vi "Counts Per Second to RPM.vi"(10 "Counts/Rev":dbl, 11 "Counts/Second":dbl) -> (3 "RPM":dbl)   [LabVIEW 2013]
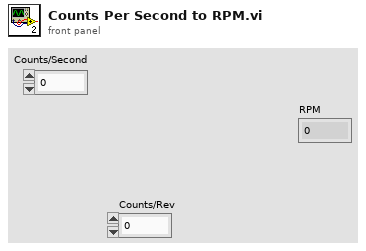
[diagram p1: front panel]
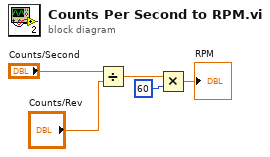
[diagram p0: block diagram]
diagram:
  n1 = Divide(x="Counts/Second", y="Counts/Rev") -> (x/y=w3:dbl)
  n2 = Multiply(x=w3, y=60) -> (x*y=→"RPM":dbl)
